vi "Get All Classes Properties and Methods.vi"(8 "error in":errorcluster) -> (0 "error out":errorcluster, 1 "Methods[]":T1(array[cluster]), 2 "Properties[]":T2(array[cluster]), 3 "Classes[]":T3(array[cluster]))   [LabVIEW 2023]
doc: "Gets all classes, properties, and methods available in LabVIEW. This is slow, as it also gets the R/W-ability, if scripting, private, etc. Best to do this once and cache the results."
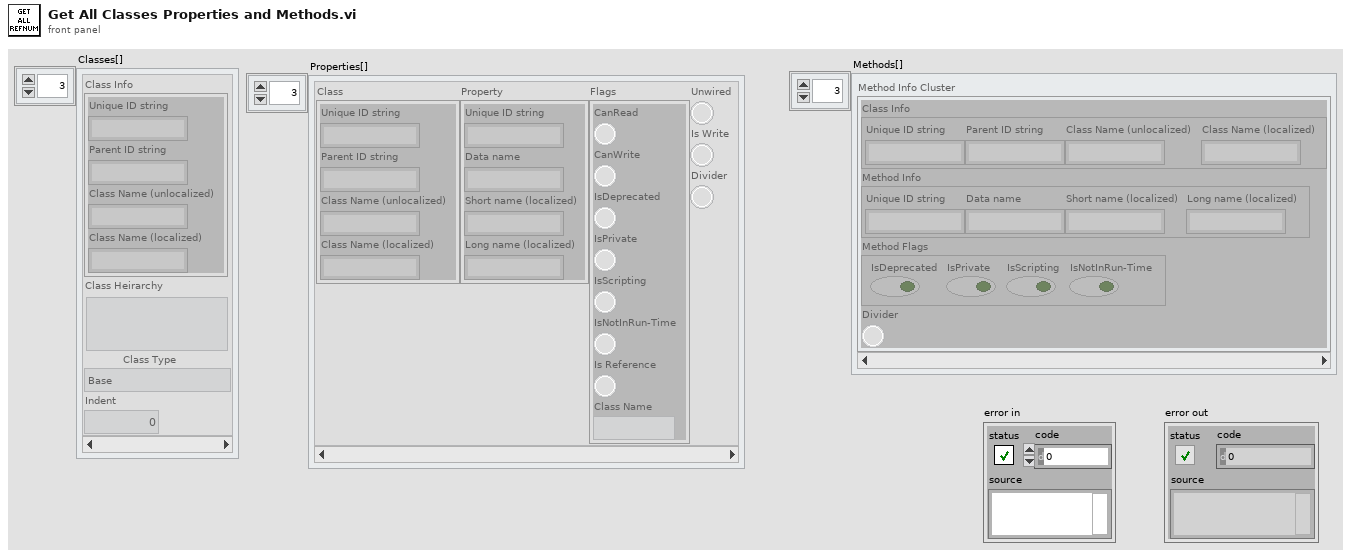
[diagram p1: front panel]
types:
  T1 = cluster{"Class Info":cluster{"Unique ID string":string, "Parent ID string":string, "Class Name (unlocalized)":string, "Class Name (localized)":string}, "Method Info":cluster{"Unique ID string":string, "Data name":string, "Short name (localized)":string, "Long name (localized)":string}, "Method Flags":cluster{"IsDeprecated":bool, "IsPrivate":bool, "IsScripting":bool, "IsNotInRun-Time":bool}, "Divider":bool}[]
  T2 = cluster{"Class":cluster{"Unique ID string":string, "Parent ID string":string, "Class Name (unlocalized)":string, "Class Name (localized)":string}, "Property":cluster{"Unique ID string":string, "Data name":string, "Short name (localized)":string, "Long name (localized)":string}, "Flags":cluster{"CanRead":bool, "CanWrite":bool, "IsDeprecated":bool, "IsPrivate":bool, "IsScripting":bool, "IsNotInRun-Time":bool, "Is Reference":bool, "Class Name":string}, "Divider":bool, "Is Write":bool, "Unwired":bool}[]
  T3 = cluster{"Class Info":cluster{"Unique ID string":string, "Parent ID string":string, "Class Name (unlocalized)":string, "Class Name (localized)":string}, "Class Heirarchy":string, "Class Type":enum16{"Unknown", "Base", "Scripting", "Private", "Deprecated", "None", "Divider"}, "Indent":u32}[]
  T4 = cluster{"Done":refnum<user-event>, "Msg 1":refnum<user-event>, "Msg 2":refnum<user-event>, "Prog Max":refnum<user-event>, "Prog Ct":refnum<user-event>}
  T5 = cluster{"Class Info":cluster{"Unique ID string":string, "Parent ID string":string, "Class Name (unlocalized)":string, "Class Name (localized)":string}, "Property Info":cluster{"Unique ID string":string, "Data name":string, "Short name (localized)":string, "Long name (localized)":string}, "Property Flags":cluster{"CanRead":bool, "CanWrite":bool, "IsDeprecated":bool, "IsPrivate":bool, "IsScripting":bool, "IsNotInRun-Time":bool, "Is Reference":bool, "Class Name":string}}[]
  T6 = cluster{"Class":cluster{"Unique ID string":string, "Parent ID string":string, "Class Name (unlocalized)":string, "Class Name (localized)":string}, "Property":cluster{"Unique ID string":string, "Data name":string, "Short name (localized)":string, "Long name (localized)":string}, "Flags":cluster{"CanRead":bool, "CanWrite":bool, "IsDeprecated":bool, "IsPrivate":bool, "IsScripting":bool, "IsNotInRun-Time":bool, "Is Reference":bool, "Class Name":string}, "Divider":bool, "Is Write":bool, "Unwired":bool}
  T7 = cluster{"Unique ID string":string, "Parent ID string":string, "Class Name (unlocalized)":string, "Class Name (localized)":string}
  T8 = cluster{"Unique ID string":string, "Data name":string, "Short name (localized)":string, "Long name (localized)":string}
  T9 = cluster{"CanRead":bool, "CanWrite":bool, "IsDeprecated":bool, "IsPrivate":bool, "IsScripting":bool, "IsNotInRun-Time":bool, "Is Reference":bool, "Class Name":string}
  T10 = cluster{"Class Info":cluster{"Unique ID string":string, "Parent ID string":string, "Class Name (unlocalized)":string, "Class Name (localized)":string}, "Method Info":cluster{"Unique ID string":string, "Data name":string, "Short name (localized)":string, "Long name (localized)":string}, "Method Flags":cluster{"IsDeprecated":bool, "IsPrivate":bool, "IsScripting":bool, "IsNotInRun-Time":bool}}[]
  T11 = cluster{"Class Info":cluster{"Unique ID string":string, "Parent ID string":string, "Class Name (unlocalized)":string, "Class Name (localized)":string}, "Method Info":cluster{"Unique ID string":string, "Data name":string, "Short name (localized)":string, "Long name (localized)":string}, "Method Flags":cluster{"IsDeprecated":bool, "IsPrivate":bool, "IsScripting":bool, "IsNotInRun-Time":bool}, "Divider":bool}
  T12 = cluster{"IsDeprecated":bool, "IsPrivate":bool, "IsScripting":bool, "IsNotInRun-Time":bool}
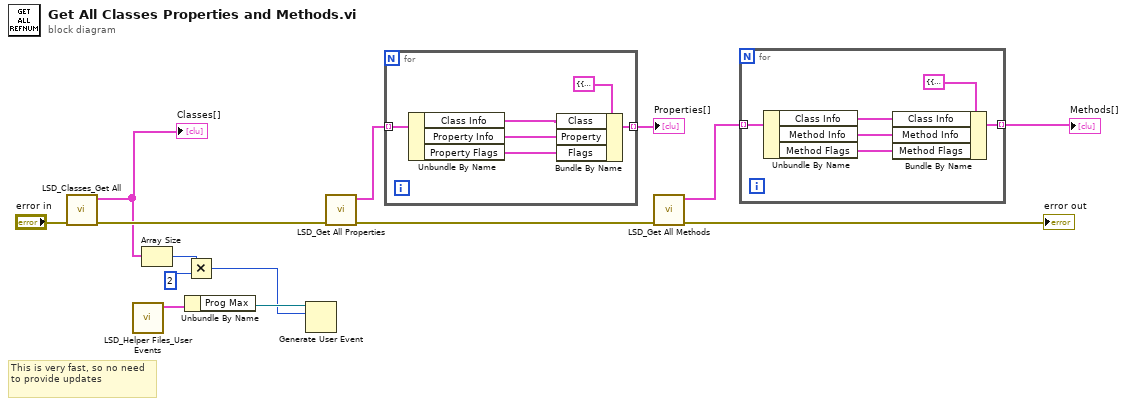
[diagram p0: block diagram]
diagram:
  # "This is very fast, so no need to provide updates"
  n1 = call <resource>:"LSD_Classes_Get All.vi"("error in"="error in") -> ("error out"=w14:errorcluster, "All Classes Tree Sorted"=w6:T3)  [unwired: 9 in]
  "Classes[]" <- w6
  n2 = call <resource>:"LSD_Helper Files_User Events.vi"() -> ("Init Dialog UEs"=w3:T4)  [unwired: 11 in]
  n3 = Array Size(array=w6) -> (size(s)=w5:i32)
  n4 = Unbundle By Name(w3) -> ("Prog Max"=w2:refnum<user-event>)
  n5 = Multiply(x=w5, y=2) -> (x*y=w1:i32)
  n6 = Generate User Event(user event=w2, event data cluster=w1) -> ()  [unwired: 2 in, 2 out]
  n7 = call <resource>:"LSD_Get All Properties.vi"("error in"=w14) -> ("error out"=w13:errorcluster, "Properties[]"=w9:T5)  [unwired: 9 in]
  n8 = for {
    tunnel: [w20] -> w10 mode=indexing
    tunnel: w9 -> [w18] mode=indexing
    n9 = Unbundle By Name(w18) -> ("Class Info"=w17:T7, "Property Info"=w16:T8, "Property Flags"=w15:T9)
    n10 = Bundle By Name(cluster=T6 {"Class"={"Unique ID string"="", "Parent ID string"="", "Class Name (unlocalized)"="", "Class Name (localized)"=""}, "Property"={"Unique ID string"="", "Data name"="", "Short name (localized)"="", "Long name (localized)"=""}, "Flags"={"CanRead"=FALSE, "CanWrite"=FALSE, "IsDeprecated"=FALSE, "IsPrivate"=FALSE, "IsScripting"=FALSE, "IsNotInRun-Time"=FALSE, "Is Reference"=FALSE, "Class Name"=""}, "Divider"=FALSE, "Is Write"=FALSE, "Unwired"=FALSE} ("Cluster"), "Class"=w17, "Property"=w16, "Flags"=w15) -> (w20:T6)
  }
  "Properties[]" <- w10
  n11 = call <resource>:"LSD_Get All Methods.vi"("error in (no error)"=w13) -> ("error out"=→"error out":errorcluster, "Methods[]"=w8:T10)  [unwired: 9 in]
  n12 = for {
    tunnel: [w26] -> w7 mode=indexing
    tunnel: w8 -> [w24] mode=indexing
    n13 = Unbundle By Name(w24) -> ("Class Info"=w23:T7, "Method Info"=w22:T8, "Method Flags"=w21:T12)
    n14 = Bundle By Name(cluster=T11 {"Class Info"={"Unique ID string"="", "Parent ID string"="", "Class Name (unlocalized)"="", "Class Name (localized)"=""}, "Method Info"={"Unique ID string"="", "Data name"="", "Short name (localized)"="", "Long name (localized)"=""}, "Method Flags"={"IsDeprecated"=FALSE, "IsPrivate"=FALSE, "IsScripting"=FALSE, "IsNotInRun-Time"=FALSE}, "Divider"=FALSE} ("Method Info Cluster"), "Class Info"=w23, "Method Info"=w22, "Method Flags"=w21) -> (w26:T11)
  }
  "Methods[]" <- w7
